vi "Get_SoftDependency.vi"(8 "error in (no error)":errorcluster, 11 "IB_SoftDependency in":refnum<class "IB_SoftDependency.lvclass">) -> (0 "error out":errorcluster, 2 "data":T1, 3 "IB_SoftDependency out":refnum<class "IB_SoftDependency.lvclass">)   [LabVIEW 2020, in "IB_SoftDependency.lvclass"]
uses:
  <vilib>/AppBuilder/IB_Classes/SoftDependency/IB_SoftDependency.lvclass
  <vilib>/AppBuilder/IB_Classes/SoftDependency/IB_SoftDependency.lvclass/IB_SoftDependency.ctl
  <vilib>/AppBuilder/IB_Classes/SoftDependency/IB_SoftDependency.ctl
  <resource>/Framework/Providers/Builds/Installer/CDK_sTypeDef_FlavorInfo.ctl
  <vilib>/AppBuilder/IB_Classes/DistPart/IB_DistPartType.ctl
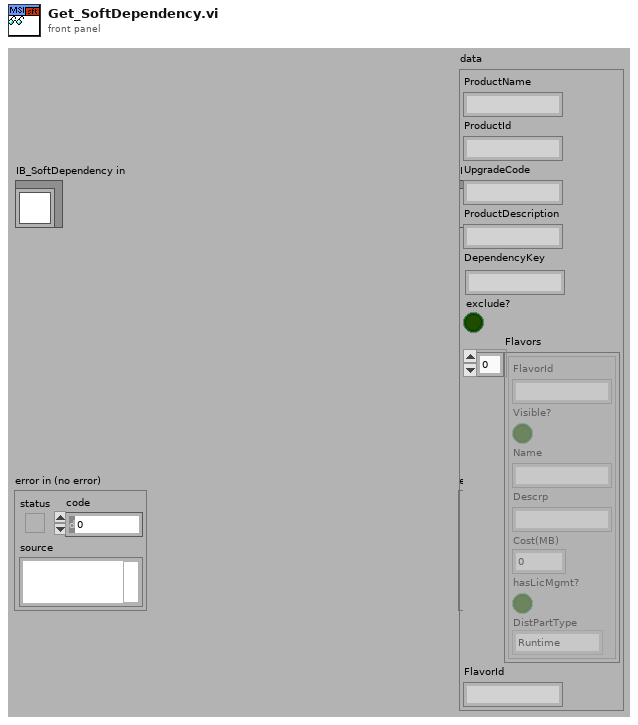
[diagram p1: front panel]
types:
  T1 = typedef "IB_SoftDependency.ctl" = cluster{"ProductName":string, "ProductId":string, "UpgradeCode":string, "ProductDescription":string, "DependencyKey":string, "exclude?":bool, "Flavors":T2[], "FlavorId":string}
  T2 = typedef "CDK_sTypeDef_FlavorInfo.ctl" = cluster{"FlavorId":string, "Visible?":bool, "Name":string, "Descrp":string, "Cost(MB)":i32, "hasLicMgmt?":bool, "DistPartType":T3}
  T3 = typedef "IB_DistPartType.ctl" = enum16{"Full", "Runtime"}
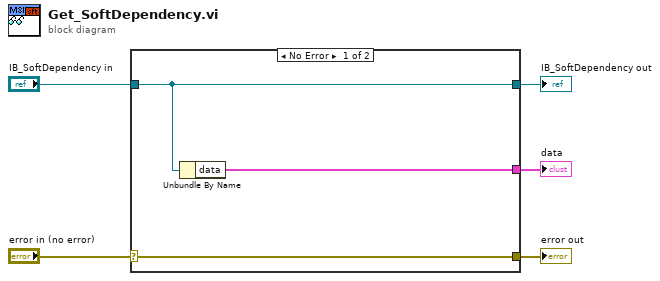
[diagram p0: block diagram]
diagram:
  n1 = case shown="No Error" "error in (no error)" {
    selector: "error in (no error)" -> [w8 w9]
    tunnel: [w8 w9] -> w4
    tunnel: [w7 w10] -> w2
    tunnel: "IB_SoftDependency in" -> [w7 w10]
    tunnel: [w6 _] -> w1
    frame No Error {
      n2 = Unbundle By Name(w7) -> ("data"=w6:T1)
    }
    frame Error {
    }
  }
  "error out" <- w4
  "IB_SoftDependency out" <- w2
  "data" <- w1
